vi "Cross Product Math.vi"(0 "Left X":dbl=15.0, 5 "Left Y":dbl=15.0, 9 "Right X":dbl=15.0, 12 "Radii (ft)":T2={"Front Left"=[11.0, 11.0, 0.0], "Front Right"=[-11.0, 11.0, 0.0], "Back Right"=[-11.0, -11.0, 0.0], "Back Left"=[11.0, -11.0, 0.0]}, 13 "Max Speed (ft/s)":dbl=15.0, 14 "Max Rotation (rad/s)":dbl) -> (6 "Modules Out":T1)   [LabVIEW 2020]
panel:
  out "BL Angle (rad)":dbl
  out "BL Velocity (ft/s)":dbl
  out "BR Angle (rad)":dbl
  out "BR Velocity (ft/s)":dbl
  out "FL Angle (rad)":dbl
  out "FL Velocity (ft/s)":dbl
  out "FR Velocity (ft/s)":dbl
  out "FR Angle (rad)":dbl
  out "Speed X":dbl=15.0
  out "Speed Y":dbl=15.0
  out "Omega":dbl[](array[numeric])
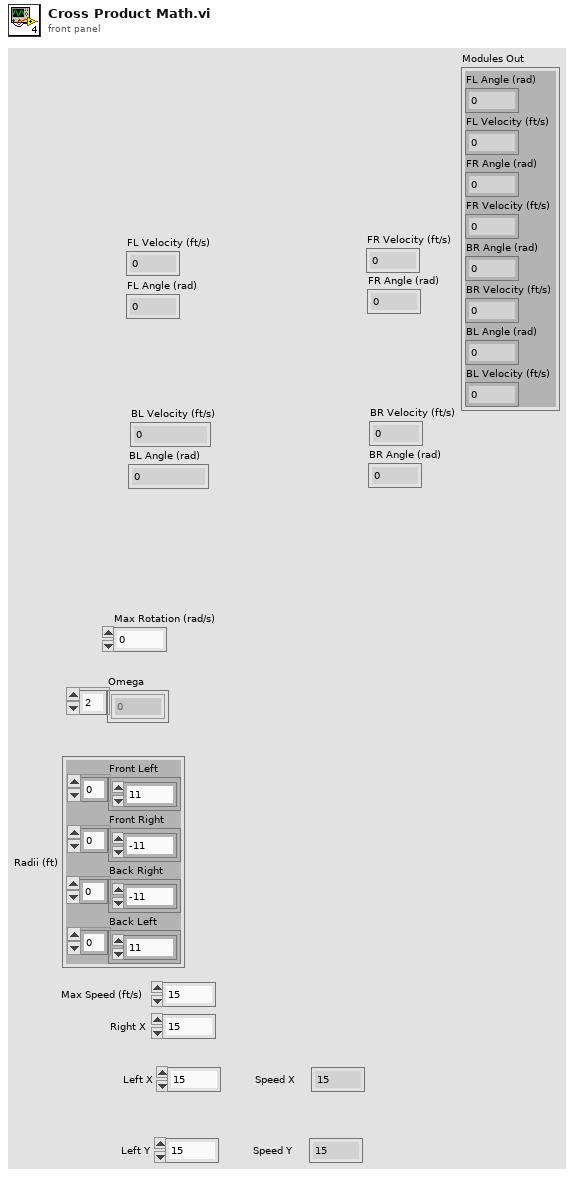
[diagram p1: front panel]
types:
  T1 = cluster{"FL Angle (rad)":dbl, "FL Velocity (ft/s)":dbl, "FR Angle (rad)":dbl, "FR Velocity (ft/s)":dbl, "BR Angle (rad)":dbl, "BR Velocity (ft/s)":dbl, "BL Angle (rad)":dbl, "BL Velocity (ft/s)":dbl}
  T2 = cluster{"Front Left":dbl[], "Front Right":dbl[], "Back Right":dbl[], "Back Left":dbl[]}
  T3 = cluster{"Speed Y":dbl, "Speed X":dbl, "Omega":dbl[]}
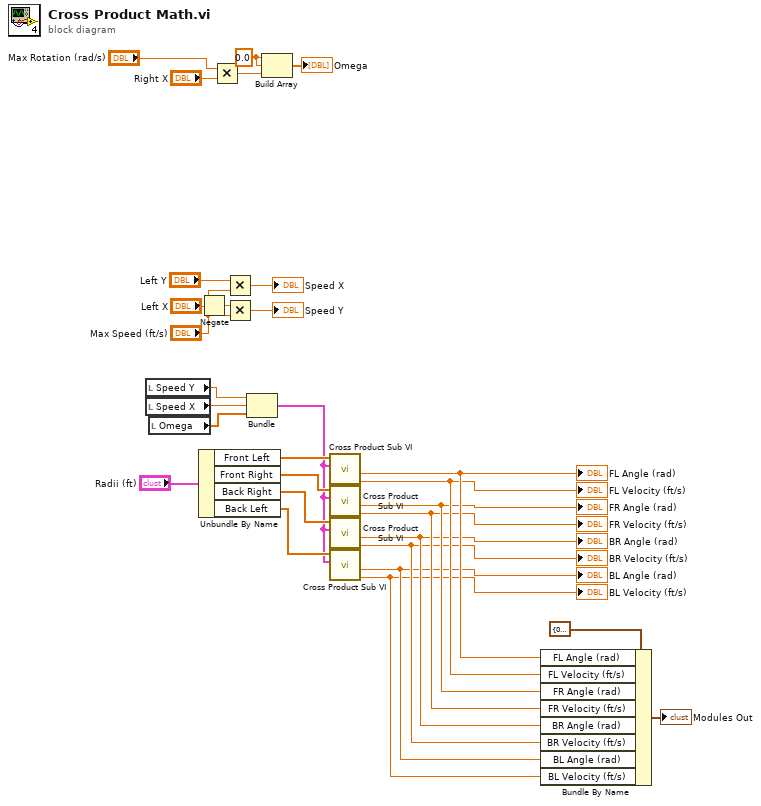
[diagram p0: block diagram]
diagram:
  w29 = 0.0 ("element")
  n1 = local read "Speed Y"() -> (w23:dbl)
  n2 = local read "Speed X"() -> (w22:dbl)
  n3 = local read "Omega"() -> (w21:dbl[])
  n4 = Negate(x="Left X") -> (-x=w4:dbl)
  n5 = Unbundle By Name("Radii (ft)") -> ("Front Left"=w20:dbl[], "Front Right"=w24:dbl[], "Back Right"=w19:dbl[], "Back Left"=w18:dbl[])
  n6 = Multiply(x="Max Rotation (rad/s)", y="Right X") -> (x*y=w25:dbl)
  n7 = Multiply(x="Left Y", y="Max Speed (ft/s)") -> (x*y=→"Speed X":dbl)
  n8 = Multiply(x=w4, y="Max Speed (ft/s)") -> (x*y=→"Speed Y":dbl)
  n9 = Bundle("Speed Y"=w23, "Speed X"=w22, "Omega"=w21) -> (w17:T3)  [unwired: 1 in]
  n10 = Build Array(w29, w29, w25) -> (→"Omega":dbl[])
  n11 = call "Cross Product Sub VI.vi"("Speed and Rotation"=w17, "Module Location"=w20) -> ("Output Velocity (ft/s)"=w15:dbl, "Output Angle (rad)"=w16:dbl)  [unwired: 5 in, 2 out]
  "FL Velocity (ft/s)" <- w15
  "FL Angle (rad)" <- w16
  n12 = call "Cross Product Sub VI.vi"("Speed and Rotation"=w17, "Module Location"=w24) -> ("Output Velocity (ft/s)"=w13:dbl, "Output Angle (rad)"=w14:dbl)  [unwired: 5 in, 2 out]
  "FR Angle (rad)" <- w14
  "FR Velocity (ft/s)" <- w13
  n13 = call "Cross Product Sub VI.vi"("Speed and Rotation"=w17, "Module Location"=w19) -> ("Output Velocity (ft/s)"=w11:dbl, "Output Angle (rad)"=w12:dbl)  [unwired: 5 in, 2 out]
  "BR Velocity (ft/s)" <- w11
  "BR Angle (rad)" <- w12
  n14 = call "Cross Product Sub VI.vi"("Speed and Rotation"=w17, "Module Location"=w18) -> ("Output Velocity (ft/s)"=w9:dbl, "Output Angle (rad)"=w10:dbl)  [unwired: 5 in, 2 out]
  "BL Velocity (ft/s)" <- w9
  "BL Angle (rad)" <- w10
  n15 = Bundle By Name(cluster=T1 {"FL Angle (rad)"=0.0, "FL Velocity (ft/s)"=0.0, "FR Angle (rad)"=0.0, "FR Velocity (ft/s)"=0.0, "BR Angle (rad)"=0.0, "BR Velocity (ft/s)"=0.0, "BL Angle (rad)"=0.0, "BL Velocity (ft/s)"=0.0} ("Module Outputs 2"), "FL Angle (rad)"=w16, "FL Velocity (ft/s)"=w15, "FR Angle (rad)"=w14, "FR Velocity (ft/s)"=w13, "BR Angle (rad)"=w12, "BR Velocity (ft/s)"=w11, "BL Angle (rad)"=w10, "BL Velocity (ft/s)"=w9) -> (→"Modules Out":T1)
